vi "InitFromXML.vi"(8 "error in (no error)":errorcluster, 10 "XML":string, 11 "Error in":refnum<class "Error.lvclass">) -> (0 "error out":errorcluster, 3 "Error out":refnum<class "Error.lvclass">)   [LabVIEW 2009, in "NavScreen.lvlib" / "Error.lvclass"]
uses:
  Error.lvclass
  ClickableText/ClickableText.lvclass
  Error.lvclass/Error.ctl
  NavScreen.lvlib
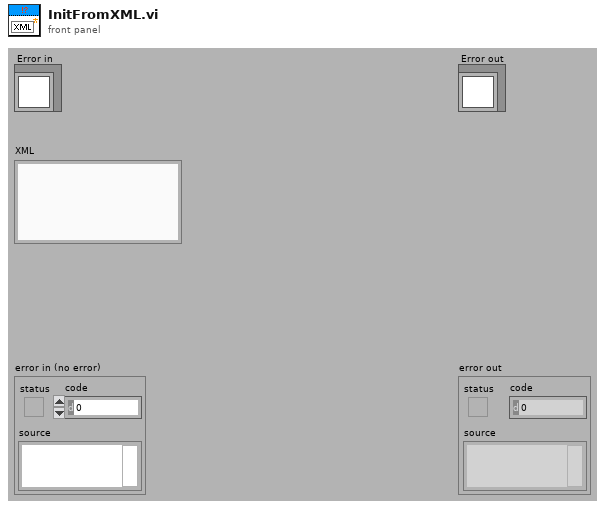
[diagram p1: front panel]
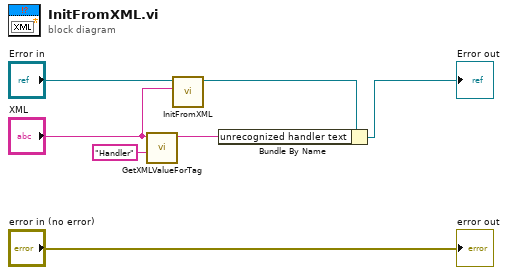
[diagram p0: block diagram]
diagram:
  n1 = call "GetXMLValueForTag.vi"("tag"="Handler", "XML"="XML") -> ("value"=w6:string)  [unwired: 8 in, 1 out]
  n2 = call-parent "InitFromXML.vi"("XML"="XML", "ClickableText in"="Error in") -> ("ClickableText out"=w2:refnum<class "Error.lvclass">)  [unwired: 8 in, 1 out]
  n3 = Bundle By Name(cluster=w2, "unrecognized handler text"=w6) -> (→"Error out":refnum<class "Error.lvclass">)
  "error out" <- "error in (no error)"
